vi "Set Log Directory.vi"(8 "error in (no error)":errorcluster, 10 "Log File Directory":path, 11 "Logger in":refnum<class "Logger.lvclass">) -> (0 "error out":errorcluster, 3 "Logger out":refnum<class "Logger.lvclass">)   [LabVIEW 2015, in "Logger Actor.lvlib" / "Logger.lvclass"]
uses:
  Logger.lvclass
  Logger.lvclass/Logger.ctl
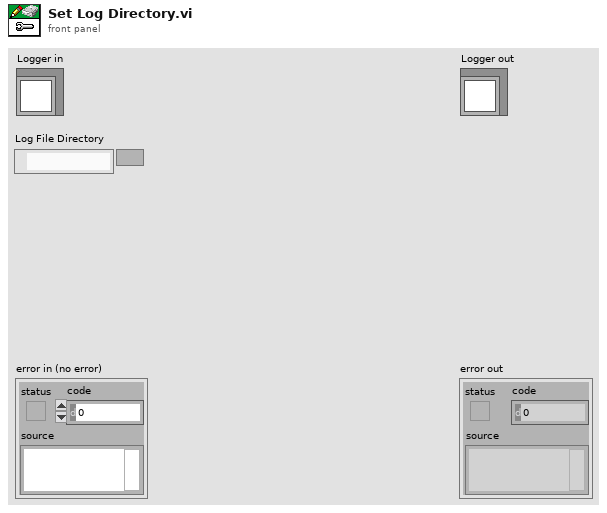
[diagram p1: front panel]
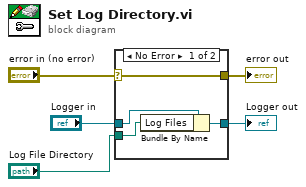
[diagram p0: block diagram]
diagram:
  n1 = case shown="No Error" "error in (no error)" {
    selector: "error in (no error)" -> [w6 w11]
    tunnel: [w6 w11] -> w4
    tunnel: [w8 w10] -> w2
    tunnel: "Logger in" -> [w9 w10]
    tunnel: "Log File Directory" -> [w7 _]
    frame No Error {
      n2 = Bundle By Name(cluster=w9, "Log Files"=w7) -> (w8:refnum<class "Logger.lvclass">)
    }
    frame Error {
    }
  }
  "error out" <- w4
  "Logger out" <- w2
